vi "Set Indicators Visibility Status.vi"(10 "Indicator Refs":refnum<vi>[](array[refnum]), 11 "Label":string) -> ()   [LabVIEW 2019, in "Panther Dashboard.lvlib"]
uses:
  Panther Dashboard.lvlib
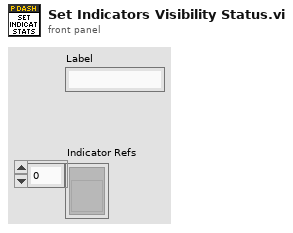
[diagram p1: front panel]
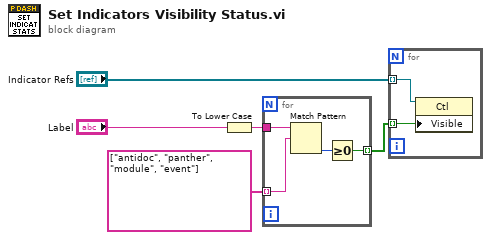
[diagram p0: block diagram]
diagram:
  n1 = To Lower Case(string="Label") -> (all lower case string=w1:string)
  n2 = for {
    tunnel: [w9] -> w5 mode=indexing
    tunnel: string[] ["antidoc", "panther", "module", "event"] ("regular expression") -> [w7] mode=indexing
    tunnel: w1 -> [w6]
    n3 = Match Pattern(string=w6, regular expression=w7) -> (offset past match=w8:i32)  [unwired: 1 in, 3 out]
    n4 = Greater Or Equal To 0?(x=w8) -> (x >= 0?=w9:bool)
  }
  n5 = for {
    tunnel: w5 -> [w11] mode=indexing
    tunnel: "Indicator Refs" -> [w10] mode=indexing
    n6 = property on="Property Node" class="Ctl"(reference=w10, "Visible"=w11) -> ()  [unwired: 1 in, 2 out]
  }
